vi "Save Embedded as File.vi"(7 "Inkscape Path":path, 8 "error in (no error)":errorcluster, 10 "Base64 Encoded String":string) -> (0 "error out":errorcluster, 2 "Path Out":string)   [LabVIEW 2019, in "SVGImage.lvclass"]
uses:
  SVGImage.lvclass
  <vilib>/LabVIEW Open Source Project/OpenSerializer.Base64/Serializer.Base64.lvclass/Serializer.Base64.ctl
  <vilib>/LabVIEW Open Source Project/OpenSerializer.Base64/Write LUT.vi
  <vilib>/LabVIEW Open Source Project/OpenSerializer.Base64/Base64_ByteLUT.vi
  <vilib>/LabVIEW Open Source Project/OpenSerializer.Base64/Decode.vi
  <vilib>/LabVIEW Open Source Project/OpenSerializer.Base64/Serializer.Base64.lvclass
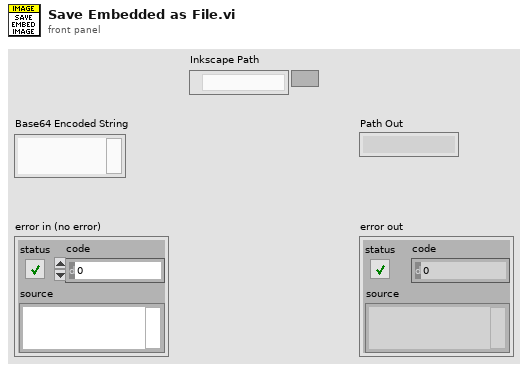
[diagram p1: front panel]
types:
  T1 = enum16{"open", "replace", "create", "open or create", "replace or create", "replace or create with confirmation"}
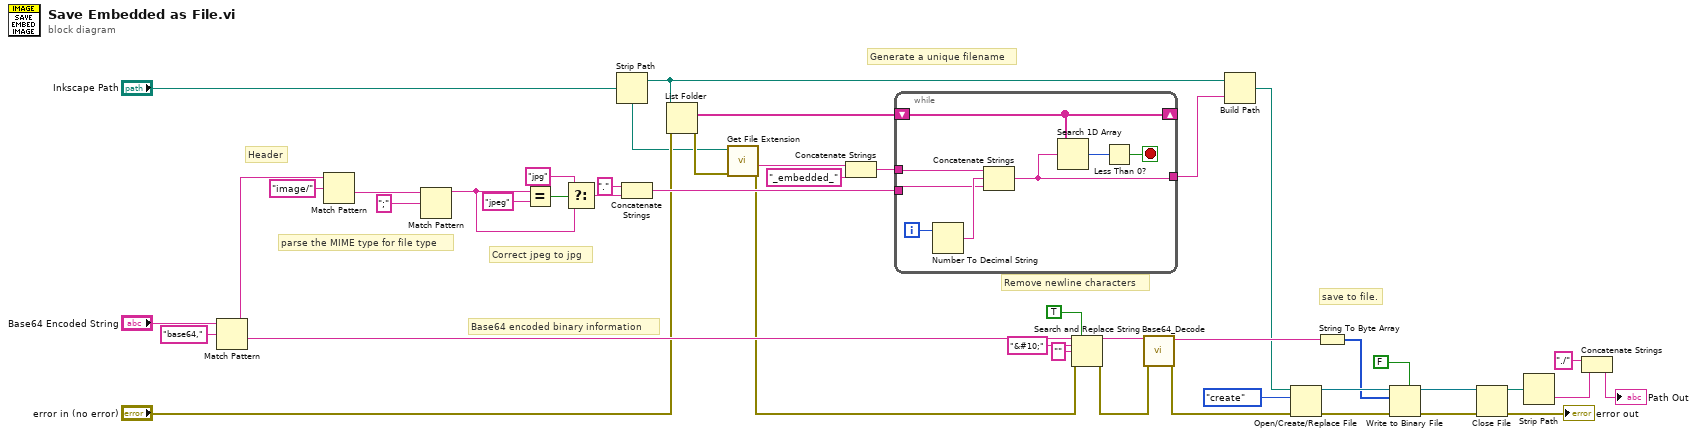
[diagram p0: block diagram]
diagram:
  # "Header"
  # "Base64 encoded binary information"
  # "Correct jpeg to jpg"
  # "parse the MIME type for file type"
  # "save to file."
  # "Remove newline characters"
  # "Generate a unique filename"
  n1 = Match Pattern(string="Base64 Encoded String", regular expression="base64,") -> (before substring=w39:string, after substring=w37:string)  [unwired: 1 in, 2 out]
  n2 = Match Pattern(string=w39, regular expression="image/") -> (after substring=w41:string)  [unwired: 1 in, 3 out]
  n3 = Match Pattern(string=w41, regular expression=";") -> (before substring=w26:string)  [unwired: 1 in, 3 out]
  n4 = Equal?(x=w26, y="jpeg") -> (x = y?=w27:bool)
  n5 = Select(t="jpg", s=w27, f=w26) -> (s? t:f=w24:string)
  n6 = Strip Path(path="Inkscape Path") -> (stripped path=w15:path)  [unwired: 1 out]
  n7 = Concatenate Strings("." ("string"), w24) -> (w22:string)
  n8 = List Folder(path=w15, error in="error in (no error)") -> (filenames=w31:string[], error out=w14:errorcluster)  [unwired: 2 in, 2 out]
  n9 = call <vilib>:"Get File Extension.vi"("error in (no error)"=w14, "file"="Inkscape Path") -> ("error out"=w13:errorcluster, "filename without extension"=w33:string)  [unwired: 5 in, 3 out]
  n10 = Concatenate Strings(w33, "_embedded_" ("string")) -> (w30:string)
  n11 = while {
    shift-right: [w46] -> _
    shift-left: w31 -> [w46]
    tunnel: w30 -> [w50]
    tunnel: w22 -> [w49]
    tunnel: [w45] -> w29
    i -> [w52]
    stop <- w47 stop-if-true
    n12 = Number To Decimal String(number=w52) -> (decimal integer string=w51:string)  [unwired: 1 in]
    n13 = Concatenate Strings(w50, w51, w49) -> (w45:string)
    n14 = Search 1D Array(1D array=w46, element=w45) -> (index of element=w48:i32)  [unwired: 1 in]
    n15 = Less Than 0?(x=w48) -> (x < 0?=w47:bool)
  }
  n16 = Search and Replace String(replace all?=TRUE ("replace all? (F)"), input string=w37, search string="&#10;", replace string="" ("replace string (\"\")"), error in=w13) -> (result string=w35:string, error out=w11:errorcluster)  [unwired: 3 in, 2 out]
  n17 = call <vilib>:"Base64_Decode.vi"("error in (no error)"=w11, "Base64 String"=w35) -> ("error out"=w12:errorcluster, "Decoded String"=w34:string)  [unwired: 8 in]
  n18 = Build Path(base path=w15, name or relative path=w29) -> (appended path=w16:path)
  n19 = Open/Create/Replace File(file path (use dialog)=w16, error in=w12, operation (0:open)=T1."create") -> (refnum out=w20:refnum<file>, error out=w18:errorcluster)  [unwired: 3 in, 1 out]
  n20 = String To Byte Array(string=w34) -> (unsigned byte array=w19:u8[])
  n21 = Write to Binary File(file (use dialog)=w20, data=w19, error in=w18, 5:FALSE ("prepend array or string size? (T)")) -> (refnum out=w17:refnum<file>, error out=w10:errorcluster)  [unwired: 2 in, 1 out]
  n22 = Close File(refnum=w17, error in=w10) -> (path=w4:path, error out=→"error out":errorcluster)
  n23 = Strip Path(path=w4) -> (name=w3:string)  [unwired: 1 out]
  n24 = Concatenate Strings("./" ("string"), w3) -> (→"Path Out":string)
